vi "Build Depends String.vi"(8 "error in (no error)":errorcluster, 10 "Build Type String":string, 11 "Dependencies Set":set{string}(c389)) -> (0 "error out":errorcluster, 3 "DEPENDS String":string)   [LabVIEW 2019, in "NIPKG Naming.lvlib"]
uses:
  NIPKG Naming.lvlib
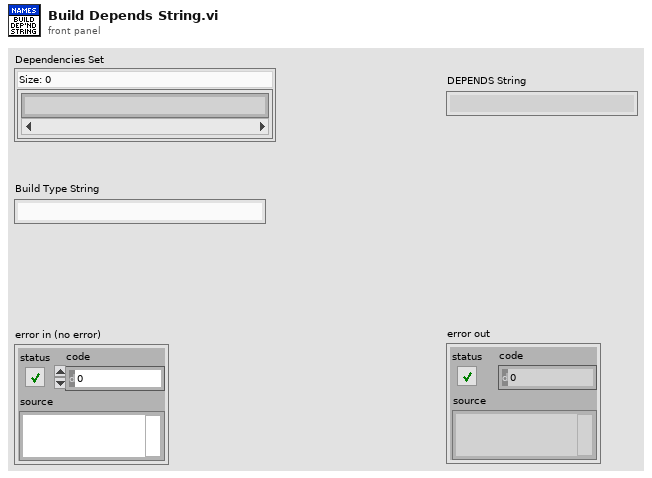
[diagram p1: front panel]
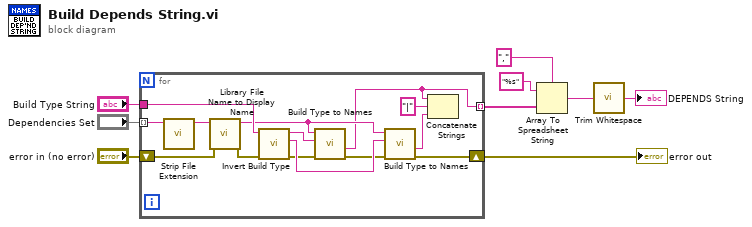
[diagram p0: block diagram]
diagram:
  n1 = for {
    tunnel: "Dependencies Set" -> [w21] mode=indexing
    tunnel: [w10] -> w8 mode=indexing
    tunnel: "Build Type String" -> [w23]
    shift-right: [w11] -> w1
    shift-left: "error in (no error)" -> [w14]
    n2 = call "Strip File Extension.vi"("LVLIBP Name In"=w21) -> ("Library Name with Extension Stripped"=w20:string)  [unwired: 10 in]
    n3 = call "Library File Name to Display Name.vi"("error in (no error)"=w14, "Library Name"=w20) -> ("error out"=w15:errorcluster, "Display Name"=w19:string)  [unwired: 8 in]
    n4 = call "Invert Build Type.vi"("error in (no error)"=w15, "Build Type String"=w23) -> ("error out"=w13:errorcluster, "Inverted Build Type"=w18:string, "Build Type String out (dup)"=w17:string)  [unwired: 7 in]
    n5 = call "Build Type to Names.vi"("error in (no error)"=w13, "Build Type String"=w17, "Library Name"=w19) -> ("error out"=w12:errorcluster, "Package Name"=w10:string)  [unwired: 5 in, 2 out]
    n6 = call "Build Type to Names.vi"("error in (no error)"=w12, "Build Type String"=w18, "Library Name"=w19) -> ("error out"=w11:errorcluster, "Package Name"=w16:string)  [unwired: 5 in, 2 out]
    n7 = Concatenate Strings(w10, "|" ("string"), w16) -> ()  [unwired: 1 out]
  }
  "error out" <- w1
  n8 = Array To Spreadsheet String(delimiter (Tab)=",", array=w8, 3:"%s" ("format string")) -> (spreadsheet string=w7:string)
  n9 = call <vilib>:"Trim Whitespace.vi"("string"=w7) -> ("trimmed string"=→"DEPENDS String":string)  [unwired: 1 in]
